vi "Read.vi"(8 "error in (no error)":errorcluster, 9 "Timeout":u32, 10 "Last message":refnum<class "BaseMessage.lvclass">, 11 "QueueReader in":refnum<class "MultiQueueReader.lvclass">) -> (0 "error out":errorcluster, 1 "isAck?":bool, 2 "Responses":T1[](array[typedef]), 3 "QueueReader out":refnum<class "MultiQueueReader.lvclass">)   [LabVIEW 2013, in "MultiQueueReader.lvclass"]
doc: "Read a message from the remote destination"
uses:
  MultiQueueReader.lvclass
  Message/BaseMessage/BaseMessage.lvclass
  response.ctl
  driver_status.ctl
  MultiQueueReader.lvclass/MultiQueueReader.ctl
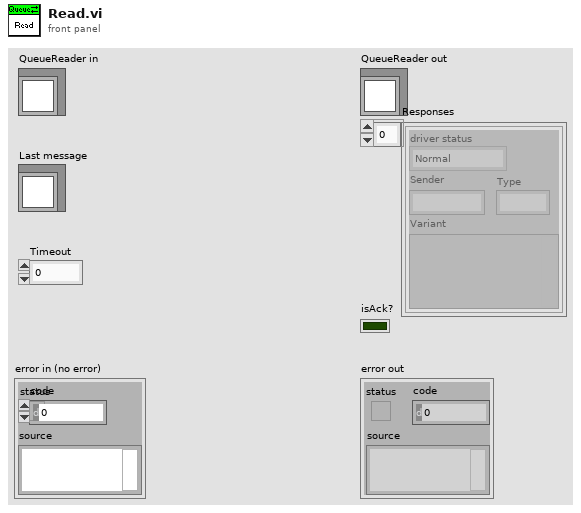
[diagram p1: front panel]
types:
  T1 = typedef "response.ctl" = cluster{"driver status":T2, "Sender":string, "Type":i32, "Variant":variant}
  T2 = typedef "driver_status.ctl" = enum16{"Normal", "Startup", "Connection lost", "Reconnected", "Timeout", "Idle", "Busy"}
  T3 = typedef "response queue.ctl" = refnum<queue>
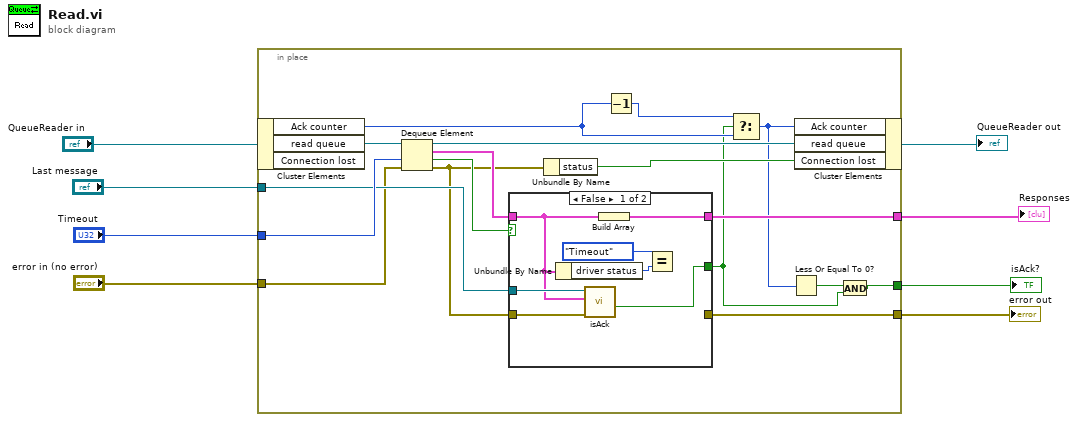
[diagram p0: block diagram]
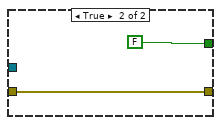
[diagram p2: hidden frame]
diagram:
  n1 = in-place "In Place Element Structure" {
    in-place-border: "Timeout" -> [w24]
    in-place-border: "Last message" -> [w22]
    in-place-border: "error in (no error)" -> [w21]
    in-place-border: [w20] -> w4
    in-place-border: [w18] -> w3
    in-place-border: [w9] -> w1
    n2 = in-place-cluster #1("QueueReader in") -> ("Ack counter"=w14:i32, "read queue"=w15:T3)  [unwired: 1 out]
    n3 = Dequeue Element(queue=w15, timeout in ms (-1)=w24, error in (no error)=w21) -> (queue out=w25:T3, element=w23:T1, timed out?=w19:bool, error out=w17:errorcluster)
    n4 = case shown="False" w19 {
      tunnel: w23 -> [w29 _]
      tunnel: w22 -> [w32 _]
      tunnel: [w26 FALSE ("isAck?")] -> w10
      tunnel: w17 -> [w31 w33]
      tunnel: [_ w33] -> w20
      tunnel: [w30 _] -> w18
      frame False {
        n5 = Unbundle By Name(w29) -> ("driver status"=w28:T2)
        n6 = call-dynamic "isAck.vi"("error in (no error)"=w31, "response"=w29, "BaseMessage in"=w32) -> ("isAck?"=w26:bool)  [unwired: 6 in, 2 out]
        n7 = Build Array(w29) -> (w30:T1[])
        n8 = Equal?(x=driver_status."Timeout", y=w28) -> ()  [unwired: 1 out]
      }
      frame True {
      }
    }
    n9 = Unbundle By Name(w17) -> ("status"=w16:bool)
    n10 = Decrement(x=w14) -> (x-1=w13:i32)
    n11 = Select(t=w13, s=w10, f=w14) -> (s? t:f=w12:i32)
    n12 = Less Or Equal To 0?(x=w12) -> (x <= 0?=w11:bool)
    n13 = in-place-cluster #1("Ack counter"=w12, "read queue"=w25, "Connection lost"=w16) -> (→"QueueReader out":refnum<class "MultiQueueReader.lvclass">)
    n14 = And(x=w11, y=w10) -> (x .and. y?=w9:bool)
  }
  "error out" <- w4
  "Responses" <- w3
  "isAck?" <- w1
